vi "LEP_RV_USBTargetError.vi"(11 "source":string) -> (3 "source out":string)   [LabVIEW 2011]
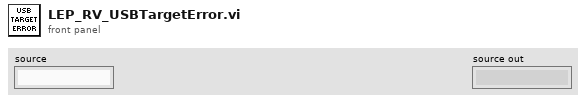
[diagram p1: front panel]
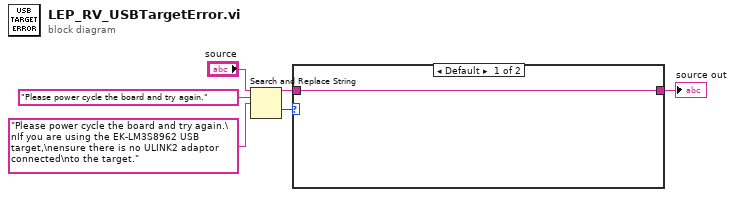
[diagram p0: block diagram]
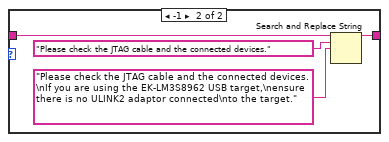
[diagram p2: hidden frame]
diagram:
  n1 = Search and Replace String(input string="source", search string="Please power cycle the board and try again.", replace string="Please power cycle the board and try again.\nIf you are using the EK-LM3S8962 USB target,\nensure there is no ULINK2 adaptor connected\nto the target." ("replace string (\"\")")) -> (result string=w3:string, offset past replacement=w4:i32)  [unwired: 5 in, 2 out]
  n2 = case shown="Default" w4 {
    tunnel: w3 -> [w7 w11]
    tunnel: [w7 w10] -> w2
    frame Default {
    }
    frame -1 {
      n3 = Search and Replace String(input string=w11, search string="Please check the JTAG cable and the connected devices.", replace string="Please check the JTAG cable and the connected devices.\nIf you are using the EK-LM3S8962 USB target,\nensure there is no ULINK2 adaptor connected\nto the target." ("replace string (\"\")")) -> (result string=w10:string)  [unwired: 5 in, 3 out]
    }
  }
  "source out" <- w2
